vi "move.vi"(8 "error in (no error)":errorcluster, 11 "Cat in":refnum<class "Cat.lvclass">) -> (0 "error out":errorcluster, 2 "message":string, 3 "Cat out":refnum<class "Cat.lvclass">)   [LabVIEW 2017, in "Cat.lvclass"]
uses:
  Cat.lvclass
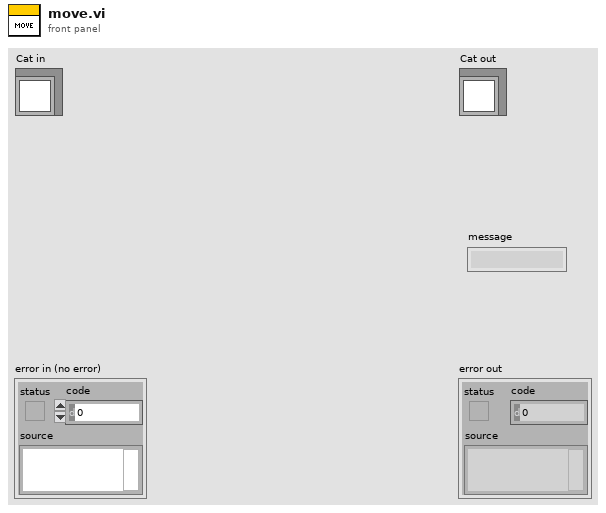
[diagram p1: front panel]
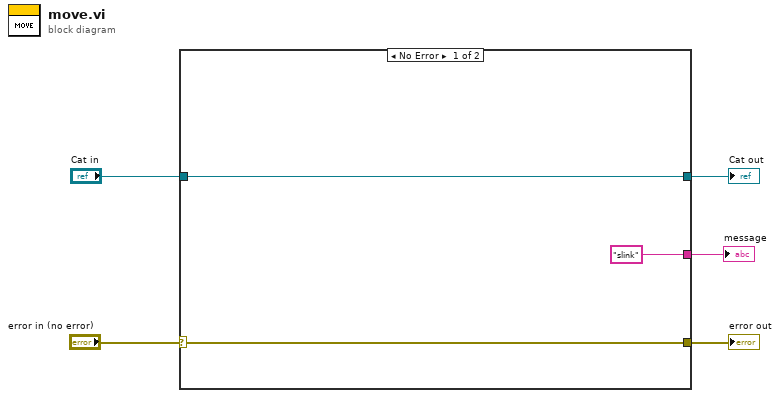
[diagram p0: block diagram]
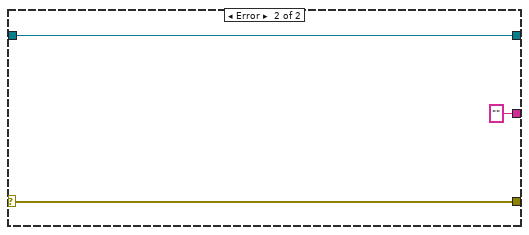
[diagram p2: hidden frame]
diagram:
  n1 = case shown="No Error" "error in (no error)" {
    selector: "error in (no error)" -> [w8 w11]
    tunnel: [w8 w11] -> w4
    tunnel: [w7 w10] -> w3
    tunnel: "Cat in" -> [w7 w10]
    tunnel: ["slink" ""] -> w1
    frame No Error {
    }
    frame Error {
    }
  }
  "error out" <- w4
  "Cat out" <- w3
  "message" <- w1
